vi "GetRefnumValue.vi"(4 "reference":refnum<class "AbstractNode.lvclass">, 5 "error in (no error)":errorcluster) -> (18 "RefNum":i32, 19 "error out":errorcluster)   [LabVIEW 2014, in "AbstractNode.lvclass"]
doc: "public Object clone()"
uses:
  <resource>/Framework/Providers/Open_GDS/UML/AbstractNode_class/AbstractNode.lvclass
  <resource>/Framework/Providers/Open_GDS/UML/AbstractNode_class/AbstractNode.lvclass/AbstractNode.ctl
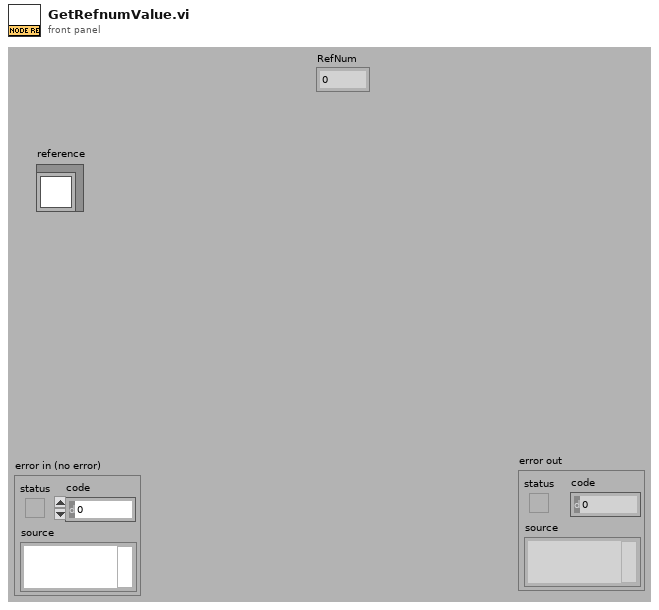
[diagram p1: front panel]
types:
  T1 = typedef "AbstractNode.lvclass/ObjectReference.ctl" = refnum<k1>
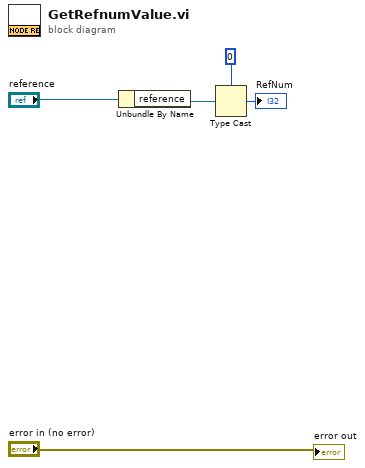
[diagram p0: block diagram]
diagram:
  n1 = Unbundle By Name("reference") -> ("reference"=w3:T1)
  n2 = Type Cast(type=0, x=w3) -> (*(type *) &x=→"RefNum":i32)
  "error out" <- "error in (no error)"
